vi "DrawSpots.vi"(7 "Spot Radius":dbl=3.0 format="%#_13g", 8 "error in (no error)":errorcluster, 9 "Draw Spots":bool, 10 "MicronsPerPx":dbl format="%#_13g", 11 "img in":T1) -> (0 "error out":errorcluster, 3 "img out":T1)   [LabVIEW 2020]
uses:
  <vilib>/vision/Image Controls.llb/IMAQ Image.ctl
  _globals/OpticalPrime Controls.vi
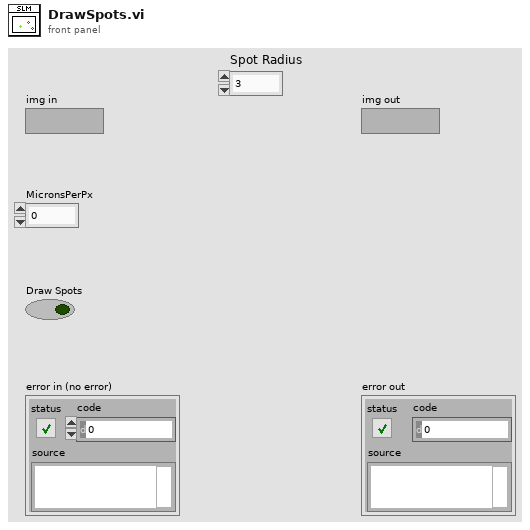
[diagram p1: front panel]
types:
  T1 = typedef "IMAQ Image.ctl" = refnum<image>
  T2 = typedef "SLM Real World to IMAQ Display Transform.ctl" = cluster{"Translation":cluster{"X":dbl, "Y":dbl}, "Scalling":cluster{"xScale":dbl, "yScale":dbl}}
  T3 = typedef "PCIe SLM Spots.ctl" = cluster{"Spot Params":T4, "Add Spot":bool, "Remove Spot":bool, "Clear All Spots":bool, "Save Spots":bool, "Generate Spots":bool, "Generate Spot Pattern":string}
  T4 = typedef "Spot Params.ctl" = cluster{"Intensity":dbl, "Vortex":dbl, "Phase":dbl, "X":dbl, "Y":dbl, "Z":dbl}[]
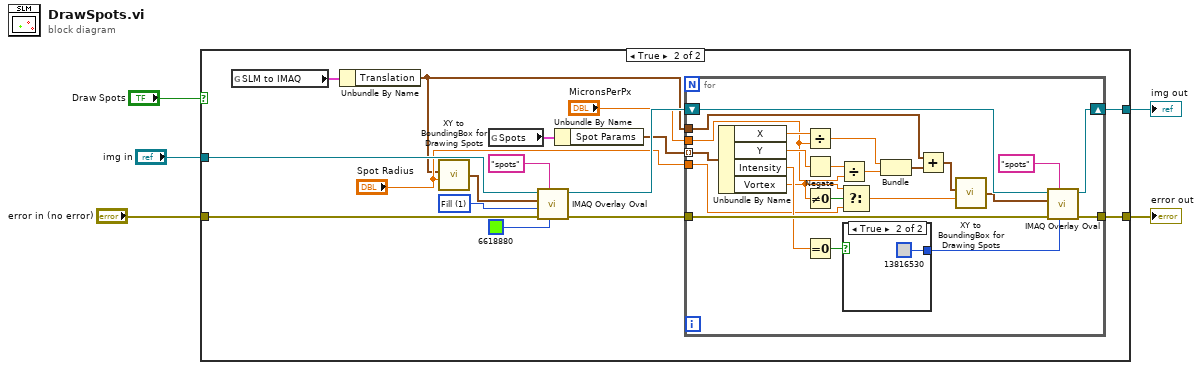
[diagram p0: block diagram]
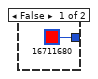
[diagram p3: hidden frame]
diagram:
  n1 = case shown="True" "Draw Spots" {
    tunnel: "img in" -> [w7 w23]
    tunnel: "error in (no error)" -> [w6 w22]
    tunnel: [w6 w16] -> w5
    tunnel: [w7 w19] -> w4
    frame False {
    }
    frame True {
      w11 = u32 1 items=["Frame", "Fill"] ("Drawing Mode (Frame)")
      n2 = global read "OpticalPrime Controls.vi" "SLM to IMAQ"() -> (w9:T2)
      n3 = Unbundle By Name(w9) -> ("Translation"=w12:cluster{"X":dbl, "Y":dbl})
      n4 = call "XY to BoundingBox for Drawing Spots.vi"("Radius"="Spot Radius", "Central Coords"=w12) -> ("Bounding Box"=w15:cluster{dbl, dbl, dbl, dbl})  [unwired: 2 in]
      n5 = global read "OpticalPrime Controls.vi" "Spots"() -> (w10:T3)
      n6 = call "IMAQ Overlay Oval"("Color"=u32 6618880, "Group"="spots", "error in (no error)"=w22, "Drawing Mode (Frame)"=w11, "Bounding Rectangle"=w15, "Image"=w23) -> ("error out"=w17:errorcluster, "Image Out"=w18:T1)  [unwired: 4 in]
      n7 = Unbundle By Name(w10) -> ("Spot Params"=w14:T4)
      n8 = for {
        tunnel: w14 -> [w44] mode=indexing
        shift-right: [w43] -> w19
        shift-left: w18 -> [w42]
        tunnel: w17 -> [w41]
        tunnel: [w40] -> w16
        tunnel: "MicronsPerPx" -> [w37]
        tunnel: w12 -> [w33]
        tunnel: "Spot Radius" -> [w25]
        n9 = Unbundle By Name(w44) -> ("X"=w39:dbl, "Y"=w38:dbl, "Intensity"=w31:dbl, "Vortex"=w26:dbl)
        n10 = Divide(x=w39, y=w37) -> (x/y=w36:dbl)
        n11 = Negate(x=w38) -> (-x=w28:dbl)
        n12 = Not Equal To 0?(x=w26) -> (x != 0?=w27:bool)
        n13 = Equal To 0?(x=w31) -> (x = 0?=w32:bool)
        n14 = Divide(x=w28, y=w37) -> (x/y=w35:dbl)
        n15 = Select(t=w26, s=w27, f=w25) -> (s? t:f=w24:dbl)
        n16 = case shown="True" w32 {
          tunnel: [u32 16711680 ("Color") u32 13816530 ("Color")] -> w46
          frame False {
          }
          frame True {
          }
        }
        n17 = Bundle(w36, w35) -> (w34:cluster{dbl, dbl})  [unwired: 1 in]
        n18 = Add(x=w33, y=w34) -> (x+y=w30:cluster{dbl, dbl})
        n19 = call "XY to BoundingBox for Drawing Spots.vi"("Radius"=w24, "Central Coords"=w30) -> ("Bounding Box"=w29:cluster{dbl, dbl, dbl, dbl})  [unwired: 2 in]
        n20 = call "IMAQ Overlay Oval"("Color"=w46, "Group"="spots", "error in (no error)"=w41, "Bounding Rectangle"=w29, "Image"=w42) -> ("error out"=w40:errorcluster, "Image Out"=w43:T1)  [unwired: 5 in]
      }
    }
  }
  "error out" <- w5
  "img out" <- w4
